vi "AudioStreamer.Init Output.vi"(0 "config":T2) -> (4 "task ID":T1 format="%.0x", 13 "framesPerStim":i32, 14 "ptsPerFrame":i32, 15 "error out":errorcluster)   [LabVIEW 2020]
uses:
  Typedefs/AudioStreamer.Config.ctl
  <vilib>/sound2/lvsound2.llb/Sound Output Task ID.ctl
  <vilib>/sound2/lvsound2.llb/Sound Data Format.ctl
  <vilib>/sound2/lvsound2.llb/Sampling Mode.ctl
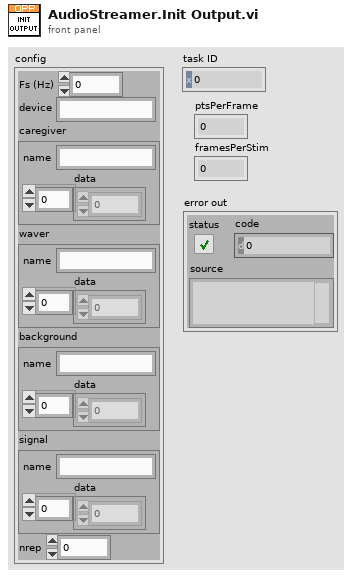
[diagram p1: front panel]
types:
  T1 = typedef "Sound Output Task ID.ctl" = u32
  T2 = typedef "AudioStreamer.Config.ctl" = cluster{"Fs (Hz)":dbl, "device":string, "caregiver":cluster{"name":string, "data":dbl[]}, "waver":cluster{"name":string, "data":dbl[]}, "background":cluster{"name":string, "data":dbl[]}, "signal":cluster{"name":string, "data":dbl[]}, "nrep":i32}
  T3 = typedef "Sound Data Format.ctl" = cluster{"sample rate (S/s)":dbl, "number of channels":i32, "bits per sample":i32}
  T4 = typedef "Sampling Mode.ctl" = i32
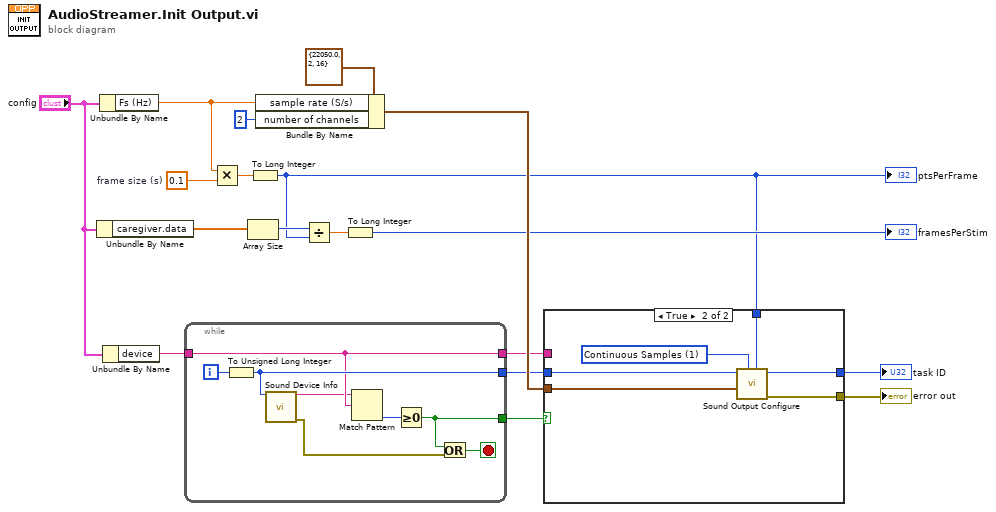
[diagram p0: block diagram]
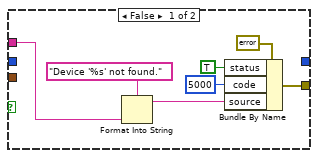
[diagram p2: hidden frame]
diagram:
  w7 = 0.1  # frame size (s)
  n1 = Unbundle By Name("config") -> ("caregiver.data"=w5:dbl[])
  n2 = Unbundle By Name("config") -> ("Fs (Hz)"=w8:dbl)
  n3 = Unbundle By Name("config") -> ("device"=w17:string)
  n4 = while {
    tunnel: w17 -> [w20]
    tunnel: [w22] -> w13
    tunnel: [w21] -> w12
    tunnel: [w20] -> w10
    i -> [w26]
    stop <- w23 stop-if-true
    n5 = To Unsigned Long Integer(number=w26) -> (unsigned 32bit integer=w22:u32)
    n6 = call <vilib>:"Sound Device Info.vi"("device"=w22) -> ("Device Name"=w19:string, "error out"=w24:errorcluster)  [unwired: 12 in, 1 out]
    n7 = Match Pattern(string=w19, regular expression=w20) -> (offset past match=w25:i32)  [unwired: 1 in, 3 out]
    n8 = Greater Or Equal To 0?(x=w25) -> (x >= 0?=w21:bool)
    n9 = Or(x=w21, y=w24) -> (x .or. y?=w23:bool)
  }
  n10 = Multiply(x=w8, y=w7) -> (x*y=w6:dbl)
  n11 = Array Size(array=w5) -> (size(s)=w4:i32)
  n12 = To Long Integer(number=w6) -> (32bit integer=w1:i32)
  "ptsPerFrame" <- w1
  n13 = Bundle By Name(cluster=T3 {"sample rate (S/s)"=22050.0, "number of channels"=2, "bits per sample"=16} ("sound format"), "sample rate (S/s)"=w8, "number of channels"=2) -> (w14:T3)
  n14 = Divide(x=w4, y=w1) -> (x/y=w3:dbl)
  n15 = To Long Integer(number=w3) -> (32bit integer=→"framesPerStim":i32)
  n16 = case shown="True" w12 {
    tunnel: [_ w39] -> w18
    tunnel: w14 -> [_ w38]
    tunnel: w13 -> [_ w37]
    tunnel: [w32 w36] -> w11
    tunnel: w10 -> [w29 _]
    tunnel: w1 -> [_ w34]
    frame False {
      n17 = Format Into String(format string="Device '%s' not found.", w29) -> (resulting string=w27:string)  [unwired: 2 in, 1 out]
      n18 = Bundle By Name(cluster=errorcluster {"status"=TRUE, "code"=5000, "source"=""} ("error out"), "status"=TRUE, "code"=5000, "source"=w27) -> (w32:errorcluster)
    }
    frame True {
      w35 = T4 1 items=["Finite Samples", "Continuous Samples"] ("sample mode")
      n19 = call <vilib>:"Sound Output Configure.vi"("number of samples/ch"=w34, "sample mode"=w35, "sound format"=w38, "device ID"=w37) -> ("error out"=w36:errorcluster, "task ID"=w39:T1)  [unwired: 6 in]
    }
  }
  "error out" <- w11
  "task ID" <- w18
